vi "Graveyard.vi"   [LabVIEW 2017, in "Tools Menu.lvlib"]
uses:
  Tools Menu.lvlib
panel:
  # "Launches the Bookmark Manager (Graveyard) dialog"
types:
  T1 = enum32{"Invalid", "Standard", "Closed", "Hidden", "Minimized", "Maximized"}
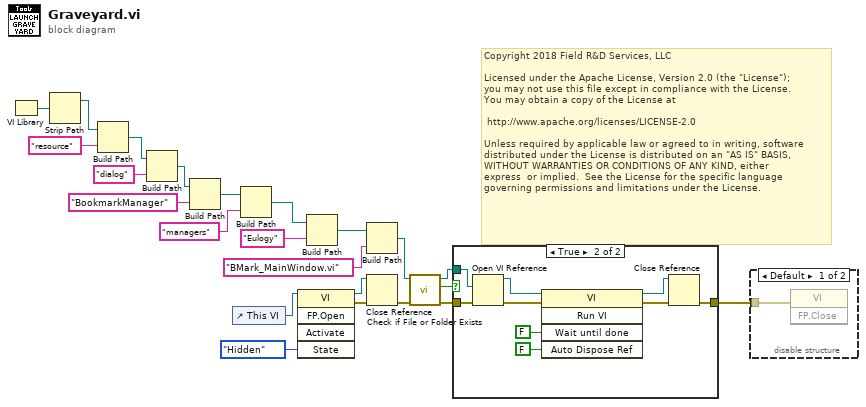
[diagram p0: block diagram]
diagram:
  # "Copyright 2018 Field R&D Services, LLC\n\nLicensed under the Apache License, Version 2.0 (the \"License\");\nyou may not use this file except in compliance with the License.\nYou may obtain a copy of the License at\n\n\thttp://www.apache.org/licenses/LICENSE-2.0\n\nUnless required by applicable law or agreed to in writing, software\ndistributed under the License is distributed on an \"AS IS\" BASIS,\nWITHOUT WARRANTIES OR CONDITIONS OF ANY KIND, either \nexpress  or implied.  See the License for the specific language \ngoverning permissions and limitations under the License."
  n1 = VI Library() -> (path=w23:path)
  n2 = Strip Path(path=w23) -> (stripped path=w22:path)  [unwired: 1 out]
  n3 = Build Path(base path=w22, name or relative path="resource") -> (appended path=w20:path)
  n4 = Build Path(base path=w20, name or relative path="dialog") -> (appended path=w18:path)
  n5 = Build Path(base path=w18, name or relative path="BookmarkManager") -> (appended path=w9:path)
  n6 = control-ref of="This VI"() -> (w5:refnum<vi>)
  n7 = Build Path(base path=w9, name or relative path="managers") -> (appended path=w7:path)
  n8 = invoke class="VI" method="FP.Open"(reference=w5, "State"=T1."Hidden") -> (reference out=w3:refnum<vi>, error out=w2:errorcluster)  [unwired: 3 in, 3 out]
  n9 = Build Path(base path=w7, name or relative path="Eulogy") -> (appended path=w15:path)
  n10 = Build Path(base path=w15, name or relative path="BMark_MainWindow.vi") -> (appended path=w13:path)
  n11 = Close Reference(reference=w3, error in (no error)=w2) -> (error out=w1:errorcluster)
  n12 = call <vilib>:"Check if File or Folder Exists.vi"("error in (no error)"=w1, "path"=w13) -> ("error out"=w10:errorcluster, "file or folder exists?"=w12:bool, "dup path"=w11:path)  [unwired: 7 in]
  n13 = case shown="True" w12 {
    tunnel: w11 -> [_ w33]
    tunnel: w10 -> [w24 w32]
    tunnel: [w24 w25] -> w6
    frame False {
    }
    frame True {
      n14 = Open VI Reference(vi path=w33, error in (no error)=w32) -> (vi reference=w31:refnum<vi>, error out=w30:errorcluster)  [unwired: 4 in]
      n15 = invoke class="VI" method="Run VI"(reference=w31, error in=w30, "Wait until done"=FALSE ("Wait Until Done"), "Auto Dispose Ref"=FALSE ("Auto Dispose Reference")) -> (reference out=w26:refnum<vi>, error out=w27:errorcluster)  [unwired: 1 in, 3 out]
      n16 = Close Reference(reference=w26, error in (no error)=w27) -> (error out=w25:errorcluster)
    }
  }
  n17 = disable-structure shown="Default" {
    disable-tunnel: w6 -> [w34 _]
    frame condition #0 {
      n18 = invoke class="VI" method="FP.Close"(error in=w34) -> ()  [unwired: 2 in, 3 out]
    }
    frame condition #1 (active) {
    }
  }
